vi "Configure Signal.vi"(7 "Signal Type (0: Voltage)":u16(ring) items=["Voltage", "Current"], 8 "error in (no error)":errorcluster, 9 "Signal Frequency (1000 Hz)":dbl=1000.0, 10 "Signal Level (1.0 V)":dbl=1.0, 11 "Agilent 428x in":refnum<class "Agilent 428x.lvclass">) -> (0 "error out":errorcluster, 3 "Agilent 428x out":refnum<class "Agilent 428x.lvclass">)   [LabVIEW 2020, in "Agilent 428x.lvclass"]
uses:
  Agilent 428x.lvclass
  C:/Sandbox/Git_Sandbox/WiSpry Test Framework source code (LV20)/WiSpry Test Framework/Instruments/Instrument.lvclass
  Instrument.lvclass/Instrument.ctl
  Instrument.lvclass
  <instrlib>/Agilent 428X Series/Agilent 428X Series.lvlib
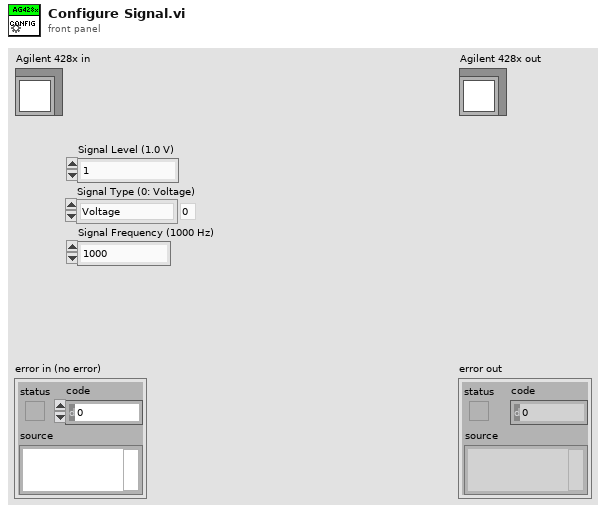
[diagram p1: front panel]
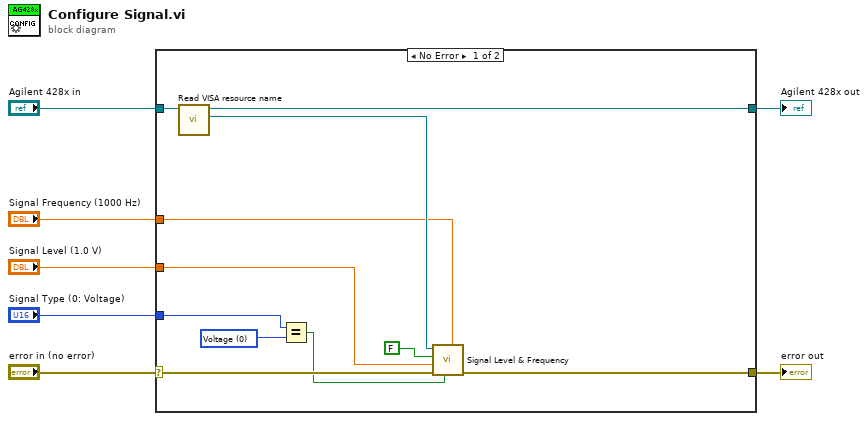
[diagram p0: block diagram]
diagram:
  n1 = case shown="No Error" "error in (no error)" {
    selector: "error in (no error)" -> [w15 w20]
    tunnel: [w14 w20] -> w6
    tunnel: [w17 w19] -> w5
    tunnel: "Agilent 428x in" -> [w18 w19]
    tunnel: "Signal Frequency (1000 Hz)" -> [w13 _]
    tunnel: "Signal Type (0: Voltage)" -> [w11 _]
    tunnel: "Signal Level (1.0 V)" -> [w9 _]
    frame No Error {
      w12 = u16 0 items=["Voltage", "Current"] ("Signal Type (0: Voltage)")
      n2 = call "Read VISA resource name.vi"("Instrument in"=w18) -> ("VISA resource name"=w16:refnum<visa-resource-name>, "Instrument out"=w17:refnum<class "Agilent 428x.lvclass">)  [unwired: 9 in]
      n3 = Equal?(x=w11, y=w12) -> (x = y?=w10:bool)
      n4 = call <instrlib>:"Signal Level & Frequency.vi"("Frequency Value (Hz) (100KHz)"=w13, "Oscillator Select (T: Voltage)"=w10, "error in (no error)"=w15, "Voltage Level (V) (5mV)"=w9, "Auto Level Control (F: Off)"=FALSE, "VISA resource name"=w16) -> ("error out"=w14:errorcluster)  [unwired: 4 in, 1 out]
    }
    frame Error {
    }
  }
  "error out" <- w6
  "Agilent 428x out" <- w5
